vi "FarfiledImageJoint.vi"() -> ()   [LabVIEW 2018]
uses:
  <vilib>/vision/NI_Vision_Development_Module.lvlib
panel:
  out "滑动杆":u8(slide) scale=0.0..128.0
  out "总时间":u32
  out "offset":i32[](array[numeric])
  out "Reference Grid":cluster{"数组":i32[], "数组":i32[]}
  out "时间":u32[](array[numeric])
  out "当前状态":cluster{"数组":i32[], "数组":i32[]}[](graph)
  out "当前图像":T1(plugin-control)
  out "总图像":T1(plugin-control)
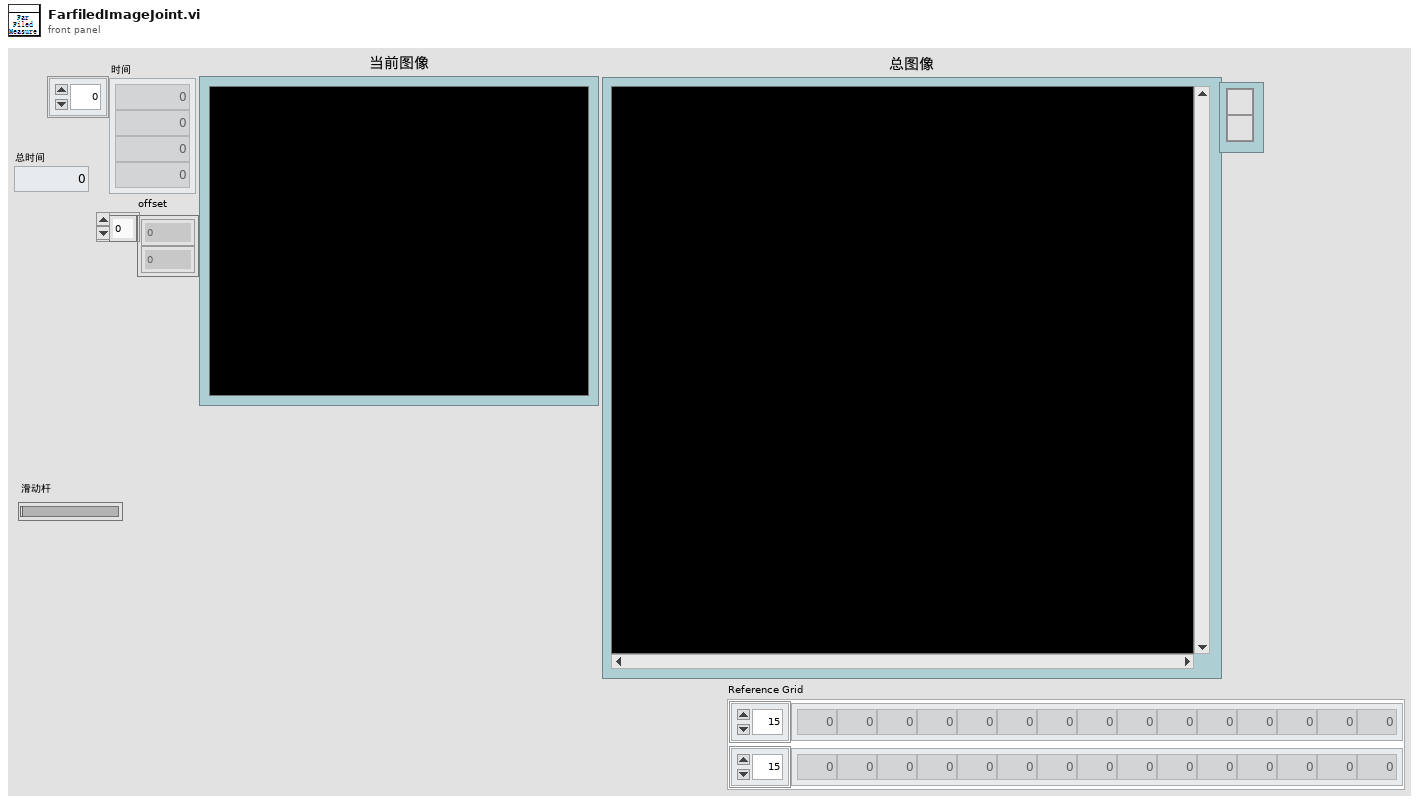
[diagram p1: front panel]
types:
  T1 = typedef "IMAQ Image.ctl" = refnum<image>
  T2 = typedef "Image Type" = u32
  T3 = typedef "控制电机枚举器.ctl" = enum16{"Z", "Y", "X", "发散角", "俯仰", "旋转"}
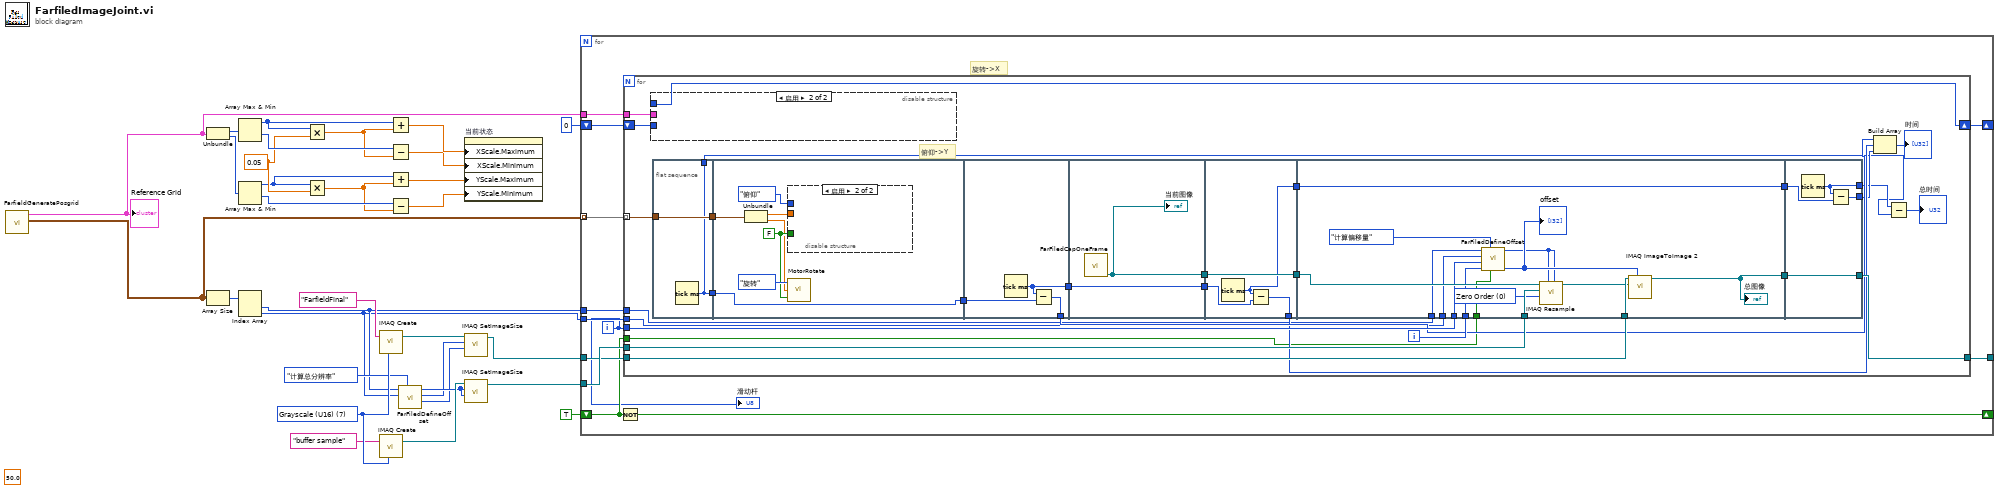
[diagram p0: block diagram]
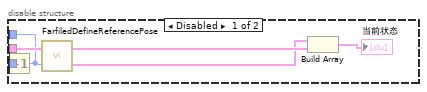
[diagram p2: hidden frame]
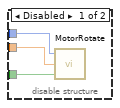
[diagram p3: hidden frame]
diagram:
  w13 = 0.05
  w27 = T2 7 items=["Grayscale (U8)", "Grayscale (I16)", "Grayscale (SGL)", "Complex (CSG)", "RGB (U32)", "HSL (U32)", "RGB (U64)", "Grayscale (U16)"] ("Image Type")
  (unwired) 50.0
  n1 = call "FarfieldGeneratePosgrid.vi"() -> ("posOut"=w31:cluster{"俯仰":dbl, "旋转":dbl}[][], "Reference Grid"=w21:cluster{"数组":i32[], "数组":i32[]})  [unwired: 9 in, 1 out]
  "Reference Grid" <- w21
  n2 = Unbundle(w21) -> ("数组"=w20:i32[], "数组"=w19:i32[])
  n3 = Array Size(array=w31) -> (size(s)=w30:i32[])
  n4 = Array Max & Min(array=w20) -> (max value=w18:i32, min value=w16:i32)  [unwired: 2 out]
  n5 = Array Max & Min(array=w19) -> (max value=w12:i32, min value=w10:i32)  [unwired: 2 out]
  n6 = Index Array(array=w30) -> (element #1=w3:i32, element #2=w2:i32)  [unwired: 2 in]
  n7 = Multiply(x=w18, y=w13) -> (x*y=w15:dbl)
  n8 = Multiply(x=w12, y=w13) -> (x*y=w9:dbl)
  n9 = call "IMAQ Create"("Image Name"="FarfieldFinal", "Image Type"=w27) -> ("New Image"=w28:T1)  [unwired: 3 in, 1 out]
  n10 = call "IMAQ Create"("Image Name"="buffer sample", "Image Type"=w27) -> ("New Image"=w25:T1)  [unwired: 3 in, 1 out]
  n11 = Add(x=w18, y=w15) -> (x+y=w17:dbl)
  n12 = Subtract(x=w16, y=w15) -> (x-y=w14:dbl)
  n13 = Add(x=w12, y=w9) -> (x+y=w11:dbl)
  n14 = Subtract(x=w10, y=w9) -> (x-y=w8:dbl)
  n15 = call "FarFiledDefineOffset.vi"("状态"=enum16{"计算总分辨率", "计算偏移量"}."计算总分辨率", "Y Pos Num"=w2, "X Pos Num"=w3) -> ("Y Resolution"=w4:i32, "X Resolution"=w5:i32, "单个分辨率"=w6:i32)  [unwired: 5 in, 1 out]
  n16 = property on="当前状态" class="XYGraph (严格)"("XScale.Maximum"=w17, "XScale.Minimum"=w14, "YScale.Maximum"=w11, "YScale.Minimum"=w8) -> ()  [unwired: 2 in, 2 out]
  n17 = call "IMAQ SetImageSize"("Y Resolution"=w4, "X Resolution"=w5, "Image"=w28) -> ("Image Out"=w23:T1)  [unwired: 2 in, 1 out]
  n18 = call "IMAQ SetImageSize"("Y Resolution"=w6, "X Resolution"=w6, "Image"=w25) -> ("Image Out"=w24:T1)  [unwired: 2 in, 1 out]
  n19 = for {
    tunnel: w31 -> [w43] mode=indexing
    tunnel: w24 -> [w42]
    shift-right: [w38] -> _
    shift-left: 0 -> [w39]
    tunnel: w21 -> [w37]
    tunnel: w3 -> [w36]
    tunnel: w2 -> [w35]
    shift-right: [w34] -> _
    shift-left: TRUE -> [w33]
    tunnel: w23 -> [w40]
    tunnel: [w41] -> _
    i -> [w32]
    # "旋转->X"
    n20 = Not(x=w33) -> (.not. x?=w34:bool)
    n21 = for {
      tunnel: w43 -> [w72] mode=indexing
      tunnel: w42 -> [w71]
      shift-right: [w66] -> w38
      shift-left: w39 -> [w68]
      tunnel: w37 -> [w67]
      tunnel: w32 -> [w64]
      tunnel: w36 -> [w59]
      tunnel: w35 -> [w58]
      tunnel: w33 -> [w57]
      tunnel: w40 -> [w69]
      tunnel: [w70] -> w41
      i -> [w65]
      # "俯仰->Y"
      n22 = disable-structure shown="启用" {
        disable-tunnel: w68 -> [w78 _]
        disable-tunnel: w67 -> [w77 _]
        disable-tunnel: [w76 _] -> w66
        frame Disabled {
          n23 = Increment(x=w78) -> (x+1=w76:i32)
          n24 = call "FarfiledDefineReferencePose.vi"("当前位置"=w76, "参考位置集合"=w77) -> ("未执行位置"=w74:cluster{"数组":i32[], "数组":i32[]}, "已经执行位置"=w75:cluster{"数组":i32[], "数组":i32[]})
          n25 = Build Array(w74, w75) -> (→"当前状态":cluster{"数组":i32[], "数组":i32[]}[])
        }
        frame Enabled {
        }
      }
      n26 = flat-sequence {
        tunnel: w72 -> [w80]
        tunnel: [w80] -> w56
        tunnel: [w79] -> w55
        tunnel: [w79] -> w45
        tunnel: w56 -> [w84]
        tunnel: w55 -> [w81]
        tunnel: [w81] -> w54
        tunnel: [w93] -> w53
        tunnel: w54 -> [w92]
        tunnel: [w91] -> w63
        tunnel: [w95] -> w52
        tunnel: w53 -> [w94]
        tunnel: [w94] -> w51
        tunnel: w52 -> [w99]
        tunnel: [w99] -> w50
        tunnel: [w97] -> w49
        tunnel: w51 -> [w98]
        tunnel: [w96] -> w62
        tunnel: w71 -> [w114]
        tunnel: w69 -> [w112]
        tunnel: w50 -> [w109]
        tunnel: w49 -> [w108]
        tunnel: [w111] -> w48
        tunnel: [w108] -> w47
        tunnel: w59 -> [w107]
        tunnel: w58 -> [w106]
        tunnel: w64 -> [w100]
        tunnel: w65 -> [w101]
        tunnel: w57 -> [w104]
        tunnel: [w118] -> w70
        tunnel: w48 -> [w118]
        tunnel: w47 -> [w117]
        tunnel: [w116] -> w61
        tunnel: [w115] -> w46
        frame #0 {
          n27 = Tick Count (ms)() -> (millisecond timer value=w79:u32)
        }
        frame #1 {
          w85 = FALSE ("是否需要测量进度？")
          n28 = Unbundle(w84) -> ("俯仰"=w83:dbl, "旋转"=w82:dbl)
          n29 = disable-structure shown="启用" {
            disable-tunnel: 控制电机枚举器."俯仰" ("控制电机") -> [w90 _]
            disable-tunnel: w85 -> [w89 _]
            disable-tunnel: w83 -> [w88 _]
            frame Disabled {
              n30 = call "MotorRotate.vi"("是否需要测量进度？"=w89, "位置"=w88, "axis"=w90) -> ()  [unwired: 1 in, 1 out]
            }
            frame Enabled {
            }
          }
          n31 = call "MotorRotate.vi"("是否需要测量进度？"=w85, "位置"=w82, "axis"=控制电机枚举器."旋转" ("控制电机")) -> ()  [unwired: 1 in, 1 out]
        }
        frame #2 {
          n32 = Tick Count (ms)() -> (millisecond timer value=w93:u32)
          n33 = Subtract(x=w93, y=w92) -> (x-y=w91:u32)
        }
        frame #3 {
          n34 = call "FarFiledCapOneFrame.vi"() -> ("Image_Normal"=w95:T1)  [unwired: 11 in]
          "当前图像" <- w95
        }
        frame #4 {
          n35 = Tick Count (ms)() -> (millisecond timer value=w97:u32)
          n36 = Subtract(x=w97, y=w98) -> (x-y=w96:u32)
        }
        frame #5 {
          w113 = u32 0 items=["Zero Order", "Bi-Linear", "Quadratic", "Cubic Spline"] ("Interpolation Type")
          n37 = call "FarFiledDefineOffset.vi"("正序？"=w104, "状态"=enum16{"计算总分辨率", "计算偏移量"}."计算偏移量", "当前Y位置"=w101, "当前X位置"=w100, "Y Pos Num"=w106, "X Pos Num"=w107) -> ("offset"=w103:i32[], "单个分辨率"=w102:i32)  [unwired: 2 in, 2 out]
          "offset" <- w103
          n38 = call "IMAQ Resample"("X Resolution"=w102, "Y Resolution"=w102, "Interpolation Type"=w113, "Image Dst"=w114, "Image Src"=w109) -> ("Image Dst Out"=w110:T1)  [unwired: 5 in, 1 out]
          n39 = call "IMAQ ImageToImage 2"("Offset Left/Top"=w103, "Image Src (Small)"=w110, "Image Src (Large)"=w112) -> ("Image Dst Out"=w111:T1)  [unwired: 7 in, 1 out]
          "总图像" <- w111
        }
        frame #6 {
          n40 = Tick Count (ms)() -> (millisecond timer value=w115:u32)
          n41 = Subtract(x=w115, y=w117) -> (x-y=w116:u32)
        }
      }
      n42 = Build Array(w63, w62, w61) -> (→"时间":u32[])
      n43 = Subtract(x=w46, y=w45) -> (x-y=→"总时间":u32)
    }
    "滑动杆" <- w32
  }
